vi "buy robots (2 resource).vi"(7 "cost of robot (X)":i32, 8 "no. robots in":i32, 9 "Y's resource in":i32, 10 "X's resource in":i32, 11 "cost of robot (Y)":i32) -> (0 "no. robots out":i32, 1 "Y's resource out":i32, 2 "X's resource out":i32)   [LabVIEW 2019]
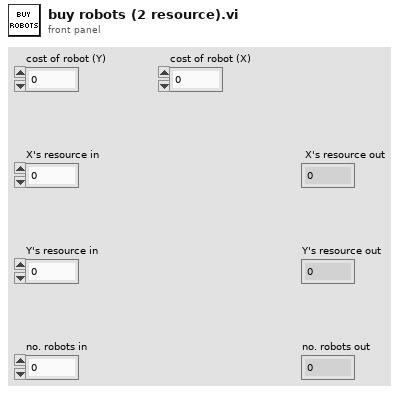
[diagram p1: front panel]
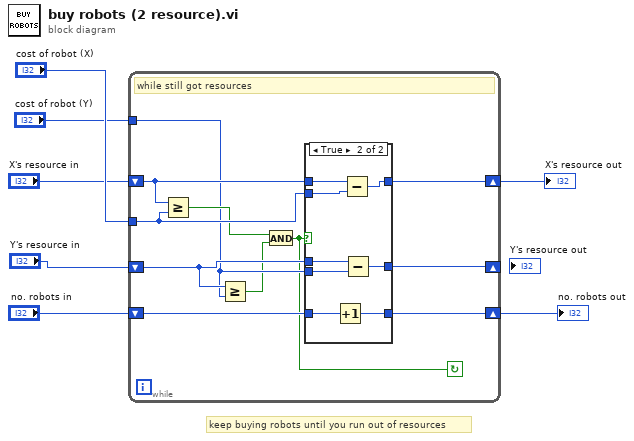
[diagram p0: block diagram]
diagram:
  # "keep buying robots until you run out of resources"
  n1 = while {
    tunnel: "cost of robot (X)" -> [w17]
    shift-right: [w18] -> w7
    shift-left: "X's resource in" -> [w16]
    shift-right: [w15] -> w4
    shift-left: "no. robots in" -> [w14]
    tunnel: "cost of robot (Y)" -> [w10]
    shift-right: [w12] -> _
    shift-left: "Y's resource in" -> [w11]
    stop <- w8 continue-if-true
    # "while still got resources"
    n2 = Greater Or Equal?(x=w16, y=w17) -> (x >= y?=w13:bool)
    n3 = Greater Or Equal?(x=w11, y=w10) -> (x >= y?=w9:bool)
    n4 = And(x=w13, y=w9) -> (x .and. y?=w8:bool)
    n5 = case shown="True" w8 {
      tunnel: [w21 w29] -> w15
      tunnel: w14 -> [w21 w28]
      tunnel: w16 -> [w20 w27]
      tunnel: w17 -> [_ w26]
      tunnel: [w20 w25] -> w18
      tunnel: w11 -> [w19 w24]
      tunnel: w10 -> [_ w23]
      tunnel: [w19 w22] -> w12
      frame False {
      }
      frame True {
        n6 = Increment(x=w28) -> (x+1=w29:i32)
        n7 = Subtract(x=w27, y=w26) -> (x-y=w25:i32)
        n8 = Subtract(x=w24, y=w23) -> (x-y=w22:i32)
      }
    }
  }
  "X's resource out" <- w7
  "no. robots out" <- w4
